vi "ReadConfig.vi"(8 "error in (no error)":errorcluster, 11 "DataLogger in":refnum<class "DataLogger.lvclass">) -> (0 "error out":errorcluster, 3 "DataLogger out":refnum<class "DataLogger.lvclass">)   [LabVIEW 2020, in "DataLogger.lvlib" / "DataLogger.lvclass"]
uses:
  DataLogger.lvclass
  DataLogger.lvclass/DataLogger.ctl
  Hardware Abstraction Layer/Component/GRMActor/GRMActor/GenericActor.lvclass
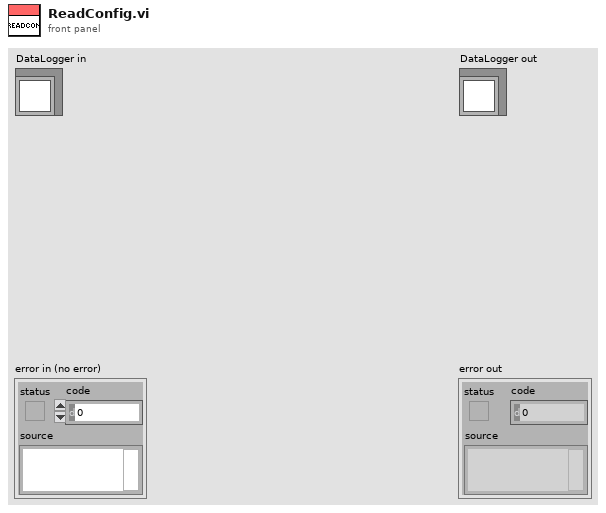
[diagram p1: front panel]
types:
  T1 = typedef "NI_LVConfig.lvlib/Config Data RefNum.ctl" = refnum<k1>
  T2 = cluster{"Values[0]":bool, "Values[1]":bool, "Values[2]":bool}
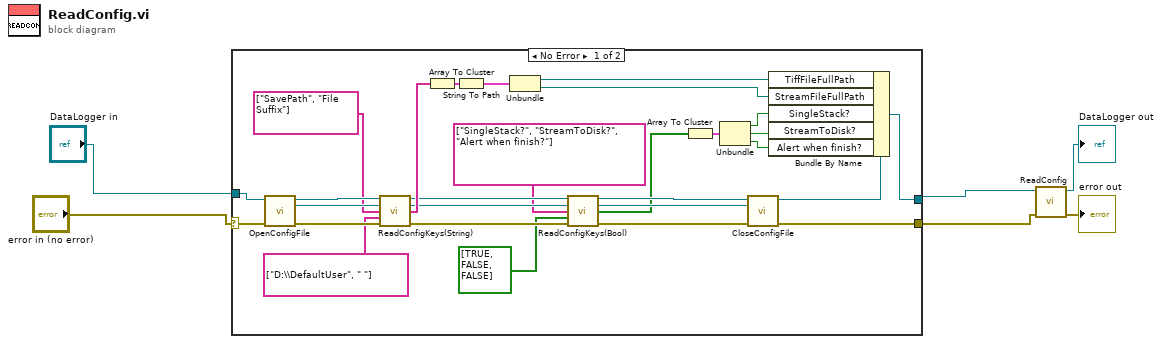
[diagram p0: block diagram]
diagram:
  n1 = case shown="No Error" "error in (no error)" {
    selector: "error in (no error)" -> [w34 w35]
    tunnel: [w27 w35] -> w1
    tunnel: [w29 w36] -> w2
    tunnel: "DataLogger in" -> [w33 w36]
    frame No Error {
      n2 = call-dynamic "OpenConfigFile.vi"("error in (no error)"=w34, "GRMActor in"=w33) -> ("error out"=w32:errorcluster, "refnum"=w28:T1, "GRMActor out"=w30:refnum<class "DataLogger.lvclass">)  [unwired: 7 in]
      n3 = call-dynamic "ReadConfigKeys(String).vi"("GRMActor in"=w30, "Config Refnum"=w28, "Keys"=string[] ["SavePath", "File Suffix"] ("Values"), "Values"=string[] ["D:\\DefaultUser", " "], "error in (no error)"=w32) -> ("GRMActor out"=w19:refnum<class "DataLogger.lvclass">, "Config Refnum dup"=w17:T1, "Values"=w25:string[], "error out"=w31:errorcluster)  [unwired: 7 in]
      n4 = Array To Cluster(array=w25) -> (cluster=w8:cluster{"Values[0]":string, "Values[1]":string})
      n5 = String To Path(string=w8) -> (path=w7:cluster{"Values[0]":path, "Values[1]":path})
      n6 = Unbundle(w7) -> ("Values[0]"=w22:path, "Values[1]"=w21:path)
      n7 = call-dynamic "ReadConfigKeys(Bool).vi"("GRMActor in"=w19, "Config Refnum"=w17, "Keys"=string[] ["SingleStack?", "StreamToDisk?", "Alert when finish?"], "Values"=bool[] [TRUE, FALSE, FALSE], "error in (no error)"=w31) -> ("GRMActor out"=w18:refnum<class "DataLogger.lvclass">, "Config Refnum dup"=w16:T1, "Values"=w13:bool[], "error out"=w20:errorcluster)  [unwired: 7 in]
      n8 = Array To Cluster(array=w13) -> (cluster=w12:T2)
      n9 = Unbundle(w12) -> ("Values[0]"=w11:bool, "Values[1]"=w10:bool, "Values[2]"=w9:bool)
      n10 = call-dynamic "CloseConfigFile.vi"("error in (no error)"=w20, "refnum"=w16, "GRMActor in"=w18) -> ("error out"=w27:errorcluster, "GRMActor out"=w26:refnum<class "DataLogger.lvclass">)  [unwired: 7 in]
      n11 = Bundle By Name(cluster=w26, "TiffFileFullPath"=w22, "StreamFileFullPath"=w21, "SingleStack?"=w11, "StreamToDisk?"=w10, "Alert when finish?"=w9) -> (w29:refnum<class "DataLogger.lvclass">)
    }
    frame Error {
    }
  }
  n12 = call-parent "ReadConfig.vi"("error in (no error)"=w1, "GRMActor in"=w2) -> ("error out"=→"error out":errorcluster, "GRMActor out"=→"DataLogger out":refnum<class "DataLogger.lvclass">)  [unwired: 8 in]
